vi "save_jt_data.vi"(4 "Intensity (no. of suns)":string, 5 "Date array":string[](array[string]), 7 "User name":string, 8 "Cell details cluster":T1={"Cell Position"=16, "Cell Label"="", "Pixel to measure"=0, "Area (cm^2)"=0.126, "Variable"="", "Variable value"="", "Scan settings in queue"=0, "Light or dark"="", "Measurement Type"=""} {"Pixel to measure" items=["All", "1", "2", "3", "4", "5", "6", "7", "8"]}, 9 "Experiment title":string) -> (1 "File path for JV data":path, 2 "File path for JV image":path)   [LabVIEW 2016]
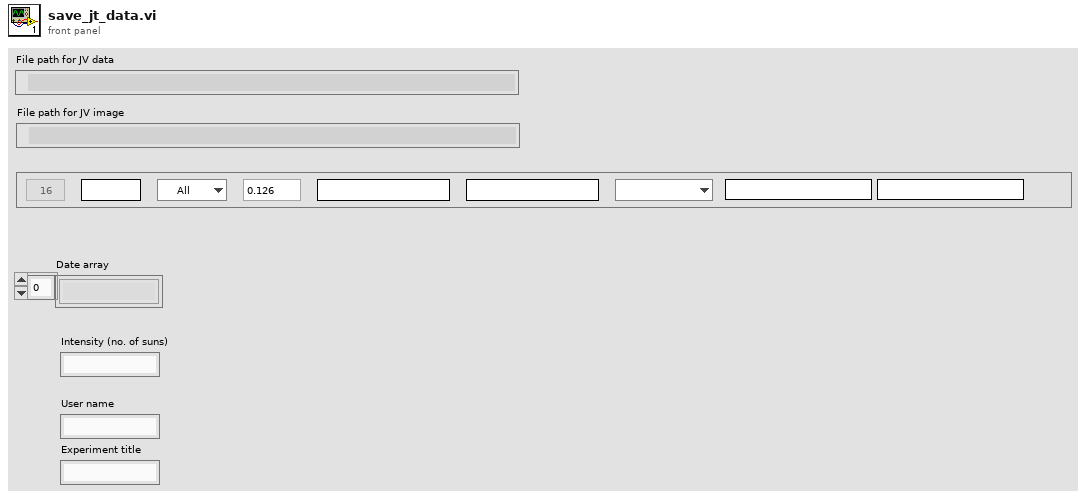
[diagram p1: front panel]
types:
  T1 = cluster{"Cell Position":i32, "Cell Label":string, "Pixel to measure":u16, "Area (cm^2)":dbl, "Variable":string, "Variable value":string, "Scan settings in queue":u16, "Light or dark":string, "Measurement Type":string}
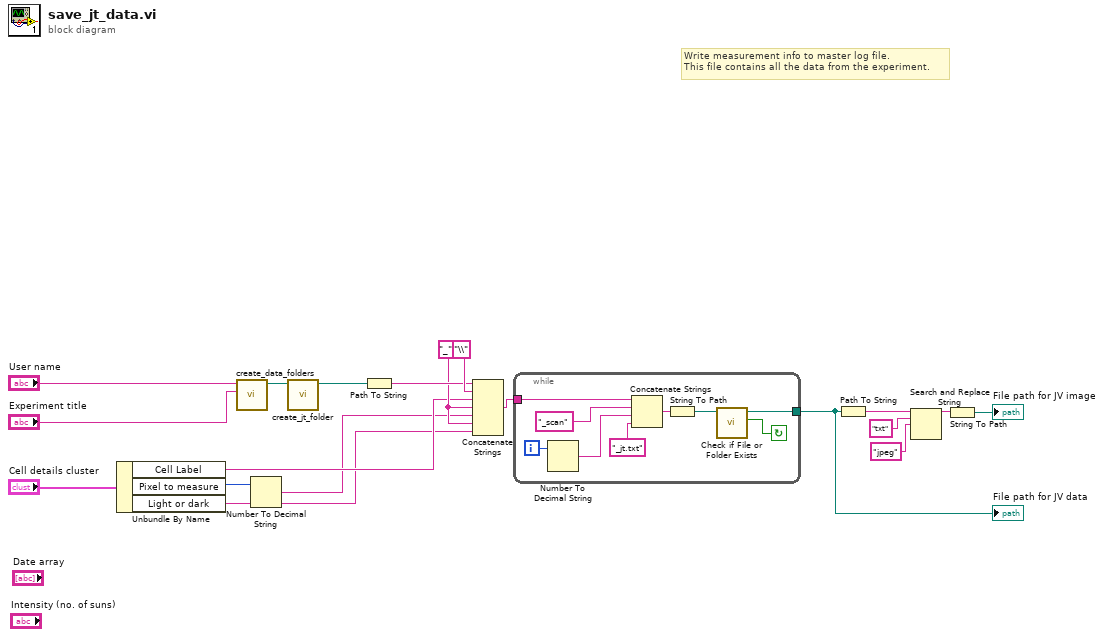
[diagram p0: block diagram]
diagram:
  w9 = "_"
  # "Write measurement info to master log file.\nThis file contains all the data from the experiment."
  n1 = Unbundle By Name("Cell details cluster") -> ("Cell Label"=w6:string, "Pixel to measure"=w4:u16, "Light or dark"=w5:string)
  n2 = call "create_data_folders.vi"("Experiment Indicator"="Experiment title", "username"="User name") -> ("Data Output Folder"=w8:path)  [unwired: 9 in]
  n3 = Number To Decimal String(number=w4) -> (decimal integer string=w3:string)  [unwired: 1 in]
  n4 = call "create_jt_folder.vi"("Data Folder In"=w8) -> ("Data Output Folder"=w7:path)  [unwired: 10 in]
  n5 = Path To String(path=w7) -> (string=w18:string)
  n6 = Concatenate Strings(w18, "\\", w6, w9, w3, w9, w5) -> (w11:string)
  n7 = while {
    tunnel: w11 -> [w28]
    tunnel: [w20] -> w1
    i -> [w26]
    stop <- w21 continue-if-true
    n8 = Number To Decimal String(number=w26) -> (decimal integer string=w25:string)  [unwired: 1 in]
    n9 = Concatenate Strings(w28, "_scan", w25, "_jt.txt") -> (w22:string)
    n10 = String To Path(string=w22) -> (path=w23:path)
    n11 = call <vilib>:"Check if File or Folder Exists.vi"("path"=w23) -> ("file or folder exists?"=w21:bool, "dup path"=w20:path)  [unwired: 8 in, 1 out]
  }
  "File path for JV data" <- w1
  n12 = Path To String(path=w1) -> (string=w10:string)
  n13 = Search and Replace String(input string=w10, search string="txt", replace string="jpeg") -> (result string=w17:string)  [unwired: 5 in, 3 out]
  n14 = String To Path(string=w17) -> (path=→"File path for JV image":path)
